vi "Write iaa.vi"(8 "error in (no error)":errorcluster, 10 "iaa":dbl[unit] min=-6.283185307179586 max=6.283185307179586, 11 "IAA.lvclass in":refnum<class "IAA.lvclass">) -> (0 "error out":errorcluster, 3 "IAA.lvclass out":refnum<class "IAA.lvclass">)   [LabVIEW 2009, in "IAA.lvclass"]
uses:
  IAA.lvclass
  IAA.lvclass/IAA.ctl
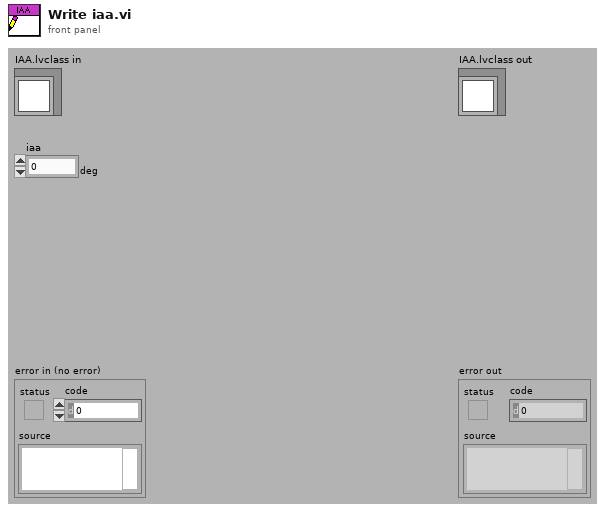
[diagram p1: front panel]
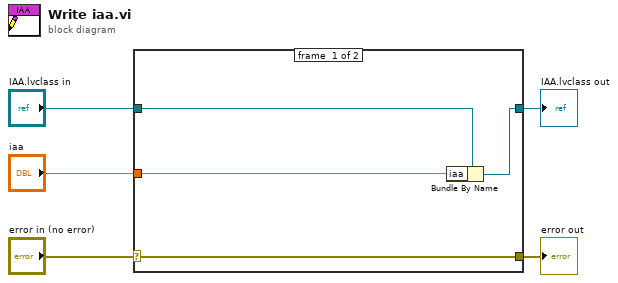
[diagram p0: block diagram]
diagram:
  n1 = case shown="No Error" "error in (no error)" {
    selector: "error in (no error)" -> [w9 w10]
    tunnel: [w9 w10] -> w4
    tunnel: [w7 w11] -> w2
    tunnel: "IAA.lvclass in" -> [w8 w11]
    tunnel: "iaa" -> [w6 _]
    frame #0 {
      n2 = Bundle By Name(cluster=w8, "iaa"=w6) -> (w7:refnum<class "IAA.lvclass">)
    }
    frame #1 {
    }
  }
  "error out" <- w4
  "IAA.lvclass out" <- w2
